vi "Posicionamento de cursores.vi"(8 "error in (no error)":errorcluster, 10 "duration":dbl, 11 "WaveformGraph in":refnum<vi>) -> (0 "error out":errorcluster)   [LabVIEW 2020]
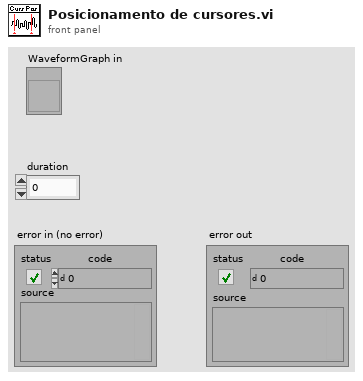
[diagram p1: front panel]
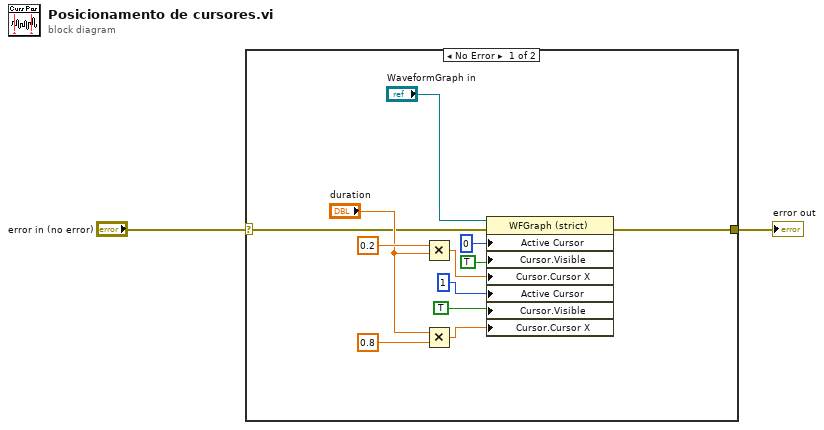
[diagram p0: block diagram]
diagram:
  n1 = case shown="No Error" "error in (no error)" {
    selector: "error in (no error)" -> [w4 w15]
    tunnel: [w3 w15] -> w1
    frame No Error {
      n2 = Multiply(x=0.2 ("y"), y="duration") -> (x*y=w5:dbl)
      n3 = Multiply(x="duration", y=0.8) -> (x*y=w6:dbl)
      n4 = property on="Property Node" class="WFGraph (strict)"(reference="WaveformGraph in", error in=w4, "Active Cursor"=u32 0, "Cursor.Visible"=TRUE, "Cursor.Cursor X"=w5, "Active Cursor"=u32 1, "Cursor.Visible"=TRUE, "Cursor.Cursor X"=w6) -> (error out=w3:errorcluster)  [unwired: 1 out]
    }
    frame Error {
    }
  }
  "error out" <- w1
